vi "SyncClassData.vi"(8 "error in (no error)":errorcluster, 11 "YActor in":refnum<class "YActor.lvclass">) -> (0 "error out":errorcluster, 3 "YActor out":refnum<class "YActor.lvclass">)   [LabVIEW 2021, in "YActor.lvclass"]
uses:
  YActor.lvclass
  SyncData.vi
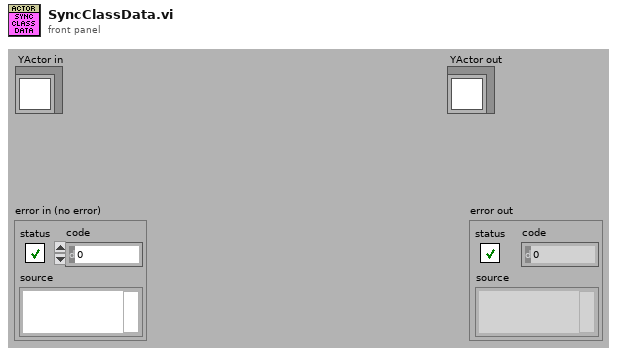
[diagram p1: front panel]
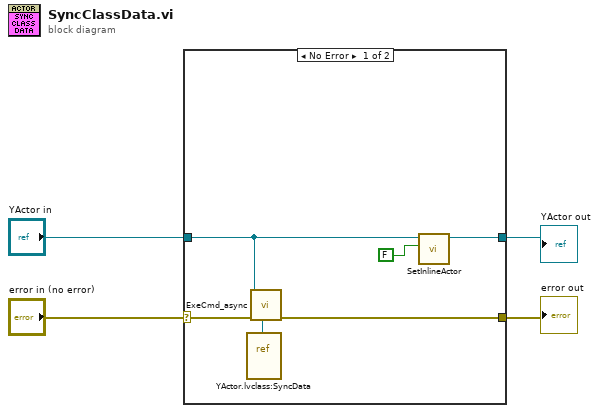
[diagram p0: block diagram]
diagram:
  n1 = case shown="No Error" "error in (no error)" {
    selector: "error in (no error)" -> [w10 w12]
    tunnel: [w9 w12] -> w3
    tunnel: "YActor in" -> [w5 w11]
    tunnel: [w7 w11] -> w1
    frame No Error {
      n2 = vi-ref "YActor.lvclass:SyncData.vi"() -> (w8:refnum<vi>)
      n3 = call "ExeCmd_async.vi"("CmdVIRef"=w8, "ErrorIn"=w10, "YActor in"=w5) -> ("ErrorOut"=w9:errorcluster)  [unwired: 8 in]
      n4 = call "SetInlineActor.vi"("Inline (T)"=FALSE ("Inline"), "YActor in"=w5) -> ("YActor out"=w7:refnum<class "YActor.lvclass">)  [unwired: 8 in, 1 out]
    }
    frame Error {
    }
  }
  "error out" <- w3
  "YActor out" <- w1
